vi "generateTelemetryIMSData.vi"(8 "error in (no error)":errorcluster, 10 "TelemetryIMSData":T1, 11 "UserEvents in":refnum<class "UserEvents.lvclass">) -> (0 "error out":errorcluster, 3 "UserEvents out":refnum<class "UserEvents.lvclass">)   [LabVIEW 2016, in "UserEvents.lvclass"]
uses:
  UserEvents.lvclass
  DataTypes/Topics/TelemetryIMSData.ctl
  DataTypes/Topics/Parts/Timestamp.ctl
  UserEvents.lvclass/UserEvents.ctl
  DataTypes/Topics/M1M3SupportTopics.lvlib
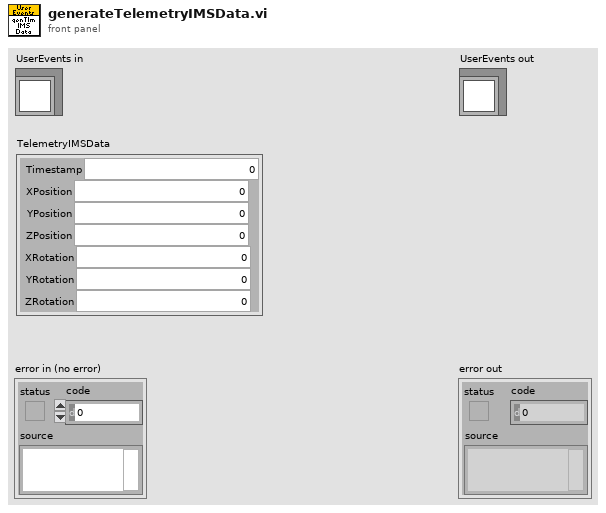
[diagram p1: front panel]
types:
  T1 = typedef "M1M3SupportTopics.lvlib/TelemetryIMSData.ctl" = cluster{"Timestamp":T2, "XPosition":dbl, "YPosition":dbl, "ZPosition":dbl, "XRotation":dbl, "YRotation":dbl, "ZRotation":dbl}
  T2 = typedef "M1M3SupportTopics.lvlib/Timestamp.ctl" = dbl
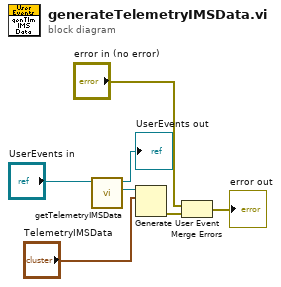
[diagram p0: block diagram]
diagram:
  n1 = call "getTelemetryIMSData.vi"("UserEvents in"="UserEvents in") -> ("TelemetryIMSData"=w7:refnum<user-event>, "UserEvents out"=→"UserEvents out":refnum<class "UserEvents.lvclass">)  [unwired: 9 in]
  n2 = Generate User Event(user event=w7, event data cluster="TelemetryIMSData") -> (error out=w4:errorcluster)  [unwired: 2 in, 1 out]
  n3 = Merge Errors("error in (no error)", w4) -> (→"error out":errorcluster)
